vi "timekeeper time rate adjust (g).vi"() -> ()   [LabVIEW 2011, in "EPS_Timekeeper.lvlib"]
uses:
  <vilib>/addons/Electrical Power/Example Support/PMU/Time Keeper/EPS_Timekeeper.lvlib
panel:
  out "time rate adjustment (g)":fxp<+/-,19,19>
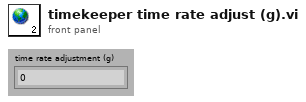
[diagram p1: front panel]
diagram:
